vi "setAndRegisterWeatherData.vi"(8 "error in (no error)":errorcluster, 10 "WeatherData.lvclass":refnum<class "WeatherData.lvclass">, 11 "CurrentConditionsDisplay in":refnum<class "DisplayBase.lvclass">) -> (0 "error out":errorcluster, 3 "CurrentConditionsDisplay out":refnum<class "DisplayBase.lvclass">)   [LabVIEW 2020]
uses:
  WeatherData/WeatherData.lvclass
  DisplayBase.lvclass
  C:/Projects/Repos/HeadFirstDesignPatterns/HeadFirstDesignPatternsLabVIEWandPython/02 Observer/LabVIEW/DisplayBase/DisplayBase.lvclass
  C:/Projects/Repos/HeadFirstDesignPatterns/HeadFirstDesignPatternsLabVIEWandPython/02 Observer/LabVIEW/DisplayElement/DisplayElement.lvclass
  C:/Projects/Repos/HeadFirstDesignPatterns/HeadFirstDesignPatternsLabVIEWandPython/02 Observer/LabVIEW/Observer/Observer.lvclass
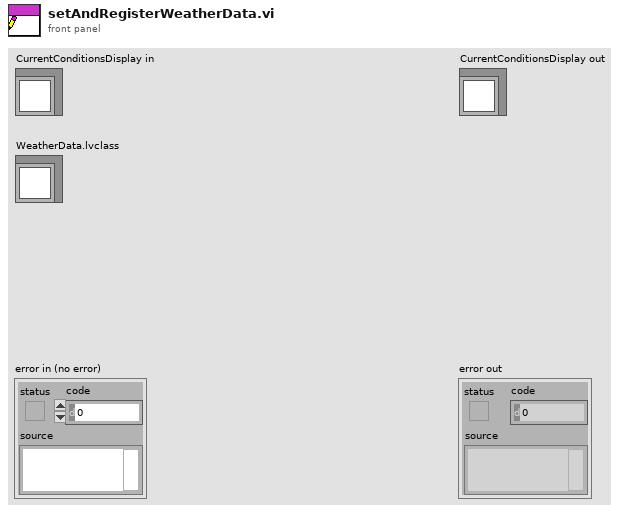
[diagram p1: front panel]
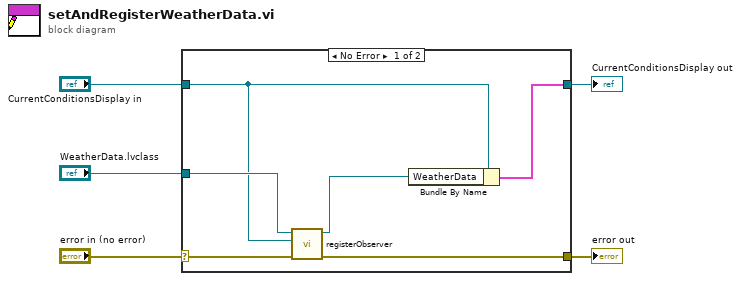
[diagram p0: block diagram]
diagram:
  n1 = case shown="No Error" "error in (no error)" {
    selector: "error in (no error)" -> [w8 w12]
    tunnel: [w7 w12] -> w4
    tunnel: [w11 w13] -> w2
    tunnel: "CurrentConditionsDisplay in" -> [w9 w13]
    tunnel: "WeatherData.lvclass" -> [w10 _]
    frame No Error {
      n2 = call-dynamic "registerObserver.vi"("error in (no error)"=w8, "Observer.lvclass"=w9, "WeatherData.lvclass"=w10) -> ("error out"=w7:errorcluster, "WeatherData.lvclass 2"=w6:refnum<class "WeatherData.lvclass">)  [unwired: 7 in]
      n3 = Bundle By Name(cluster=w9, "WeatherData"=w6) -> (w11:cluster{})
    }
    frame Error {
    }
  }
  "error out" <- w4
  "CurrentConditionsDisplay out" <- w2
